vi "UHR-Fleezers Control (host) - 12.2.vi"() -> ()   [LabVIEW 2012] (continued)
            n2466 = VISA Write(VISA resource name=w4106, write buffer=w4105) -> (VISA resource name out=w4102:refnum<visa-resource-name>)  [unwired: 1 in, 2 out]
            n2467 = Concatenate Strings("cvolume" ("string"), "\r") -> (w4103:string)
            n2468 = VISA Write(VISA resource name=w4102, write buffer=w4103) -> (VISA resource name out=w4097:refnum<visa-resource-name>)  [unwired: 1 in, 2 out]
            n2469 = Concatenate Strings("wrun" ("string"), "\r") -> (w4098:string)
            n2470 = VISA Write(VISA resource name=w4097, write buffer=w4098) -> ()  [unwired: 1 in, 3 out]
          }
        }
      }
      event "Flip Green Filter": Value Change {
        n2471 = event-data() -> ()  [unwired: 7 out]
        n2472 = Not(x="Flip Green Filter") -> (.not. x?=w4116:bool)
        n2473 = local write "Flip Green Filter"(w4116) -> ()
        n2474 = flat-sequence {
          tunnel: w4124 -> [w4129]
          tunnel: w4123 -> [w4128]
          tunnel: [w4126] -> w4121
          tunnel: [w4125] -> w4120
          tunnel: [w4131] -> w4119
          tunnel: w4121 -> [w4131]
          tunnel: [w4130] -> w4118
          tunnel: w4120 -> [w4130]
          tunnel: w4119 -> [w4135]
          tunnel: w4118 -> [w4134]
          tunnel: [w4133] -> w4122
          frame #0 {
            n2475 = xnode "Read/Write Control"("FPGA VI Reference In"=w4129, "error in"=w4128, "Green Filter Flipper"=TRUE) -> ("FPGA VI Reference Out"=w4126:T19, "error out"=w4125:errorcluster)
          }
          frame #1 {
            n2476 = Wait (ms)(milliseconds to wait=u32 100) -> ()  [unwired: 1 out]
          }
          frame #2 {
            n2477 = xnode "Read/Write Control"("FPGA VI Reference In"=w4135, "error in"=w4134, "Green Filter Flipper"=FALSE) -> ("error out"=w4133:errorcluster)  [unwired: 1 out]
          }
        }
      }
      event "Pump 1 contents", "Pump 3 contents": Value Change {
        n2478 = event-data() -> ()  [unwired: 7 out]
        n2479 = local read "Pump 1 contents"() -> (→"Pump 1 cont disp":string)
        n2480 = local read "Pump 3 contents"() -> (→"Pump 3 cont disp":string)
      }
      event "Reset Trap Pos. FB": Value Change {
        n2481 = event-data() -> ()  [unwired: 7 out]
        n2482 = xnode "Read/Write Control"("FPGA VI Reference In"=w4141, "error in"=w4140, "Trap Pos. FB Reset"="Reset Trap Pos. FB") -> ()  [unwired: 2 out]
      }
      event "Rem fb disp offset": Value Change {
        n2483 = event-data() -> ()  [unwired: 7 out]
        n2484 = local write "Rem fb disp offset"(FALSE ("Rem fb disp offset")) -> ()
        n2485 = local read "Mean T1 Position (nm)"() -> (w4143:dbl)
        n2486 = local read "FB Trap Pos Offset"() -> (w4144:dbl)
        n2487 = Subtract(x=w4144, y=w4143) -> (x-y=w4142:dbl)
        n2488 = local write "FB Trap Pos Offset"(w4142) -> ()
      }
      event "Threshold (nm)": Value Change {
        n2489 = event-data() -> ()  [unwired: 7 out]
        n2490 = flat-sequence {
          tunnel: w4148 -> [w4156]
          tunnel: w4147 -> [w4155]
          tunnel: [w4149] -> w4146
          tunnel: w4146 -> [w4162]
          frame #0 {
            n2491 = xnode "Read/Write Control"("FPGA VI Reference In"=w4156, "error in"=w4155) -> ("FPGA VI Reference Out"=w4152:T19, "error out"=w4151:errorcluster, "FPGA TTrig Thresh"=w4153:i64)
            n2492 = local read "Threshold stored (nm)"() -> (w4161:dbl)
            n2493 = local read "Threshold (nm)"() -> (w4149:dbl)
            n2494 = local read "AOM X Cal (nm/MHz)"() -> (w4159:dbl)
            n2495 = Subtract(x=w4149, y=w4161) -> (x-y=w4160:dbl)
            n2496 = Divide(x=w4160, y=w4159) -> (x/y=w4157:dbl)
            n2497 = call "IR AOM freq to word.vi"("Frequency In (MHz)"=w4157) -> ("Frequency Word Out (double)"=w4158:dbl)
            n2498 = To Quad Integer(1:w4158) -> (0:w4154:i64)
            n2499 = Add(x=w4153, y=w4154) -> (x+y=w4150:i64)
            n2500 = xnode "Read/Write Control"("FPGA VI Reference In"=w4152, "error in"=w4151, "FPGA TTrig Thresh"=w4150) -> ()  [unwired: 2 out]
          }
          frame #1 {
            "Threshold stored (nm)" <- w4162
          }
        }
      }
      event "FB Trig Integrate": Value Change {
        n2501 = event-data() -> ()  [unwired: 7 out]
        n2502 = local read "FB Trig Integrate"() -> (w4164:u32)
        n2503 = xnode "Read/Write Control"("FPGA VI Reference In"=w4166, "error in"=w4165, "FB Trig Integrate"=w4164) -> ("error out"=w4163:errorcluster)  [unwired: 1 out]
      }
      event "11": Value Change {
        n2504 = event-data() -> ()  [unwired: 7 out]
        n2505 = local read "11"() -> (w4167:bool)
        n2506 = case shown="True" w4167 {
          frame False {
          }
          frame True {
            n2507 = local read "Messages"() -> (w4169:string)
            n2508 = call "Update messages.vi"("Message to add"="You kicked it up to 11!", "Old message string"=w4169) -> ("New message string"=w4170:string)
            n2509 = call <vilib>:"Beep.vi"() -> ()  [unwired: 12 in]
            n2510 = local write "Messages"(w4170) -> ()
          }
        }
      }
      event "Trap Pos. FB ON": Value Change {
        n2511 = event-data() -> ()  [unwired: 7 out]
        n2512 = xnode "Read/Write Control"("FPGA VI Reference In"=w4173, "error in"=w4172, "Force feedback"="Trap Pos. FB ON") -> ()  [unwired: 2 out]
      }
      event "Remove Action Offset": Value Change {
        n2513 = event-data() -> ()  [unwired: 7 out]
        n2514 = local write "Remove Action Offset"(FALSE ("Remove Action Offset")) -> ()
        n2515 = local read "Trap Pos. FB Mult Factor"() -> (w4178:i64)
        n2516 = local read "Trap Pos FB Action"() -> (w4176:i64)
        n2517 = local read "Trap Pos. FB Offset Factor"() -> (w4174:i64)
        n2518 = Multiply(x=w4178, y=w4176) -> (x*y=w4177:i64)
        n2519 = Add(x=w4177, y=w4174) -> (x+y=w4175:i64)
        n2520 = local write "Trap Pos. FB Offset Factor"(w4175) -> ()
        n2521 = xnode "Read/Write Control"("FPGA VI Reference In"=w4181, "error in"=w4180, "Trap Pos. FB Offset Factor"=w4175) -> ()  [unwired: 2 out]
      }
      event "Remove Unwinding Offset": Value Change {
        n2522 = event-data() -> ()  [unwired: 7 out]
        n2523 = local write "Remove Unwinding Offset"(FALSE ("Remove Action Offset")) -> ()
        n2524 = local read "Trap Pos. FB Mult Factor"() -> (w4193:i64)
        n2525 = local read "Trap Pos FB Action"() -> (w4191:i64)
        n2526 = local read "Trap Pos. FB Offset Factor"() -> (w4190:i64)
        n2527 = Multiply(x=w4193, y=w4191) -> (x*y=w4192:i64)
        n2528 = local read "Trap Pos. FB Mult Factor"() -> (w4189:i64)
        n2529 = Add(x=w4192, y=w4190) -> (x+y=w4183:i64)
        n2530 = Multiply(x=32768, y="factor") -> (x*y=w4186:dbl)
        n2531 = Multiply(x=w4186, y=w4189) -> (x*y=w4188:dbl)
        n2532 = Subtract(x=w4183, y=w4188) -> (x-y=w4187:dbl)
        n2533 = To Quad Integer(1:w4187) -> (0:w4182:i64)
        n2534 = xnode "Read/Write Control"("FPGA VI Reference In"=w4196, "error in"=w4195, "Trap Pos. FB Offset Factor"=w4182) -> ()  [unwired: 2 out]
        n2535 = local write "Trap Pos. FB Offset Factor"(w4182) -> ()
      }
      event "Trap Pos. FB Range", "Trap Pos. FB Gains", "Trap Pos. FB Mult Factor", "Trap Pos. FB Offset Factor", "Trap Pos FB Negate Action", "Trap Pos FB Monitor\nT1 or T2", "Differential FB?", "Negate Diff?": Value Change {
        n2536 = event-data() -> ()  [unwired: 7 out]
        n2537 = Unbundle By Name("Trap Pos. FB Gains") -> ("proportional gain (Kc)"=w4199:fxp<+/-,16,8>, "integral gain (Kc*Ts/Ti)"=w4198:fxp<+/-,16,8>, "derivative gain (Kc*Td/Ts)"=w4197:fxp<+/-,16,8>)
        n2538 = local read "Negate Diff?"() -> (w4204:bool)
        n2539 = Unbundle By Name("Trap Pos. FB Range") -> ("output high"=w4202:fxp<+/-,16,1>, "output low"=w4201:fxp<+/-,16,1>)
        n2540 = xnode "Read/Write Control"("FPGA VI Reference In"=w4212, "error in"=w4211, "FB2 output high"=w4202, "FB2 output low"=w4201, "P2"=w4199, "I2"=w4198, "D2"=w4197, "Trap Pos. FB Mult Factor"="Trap Pos. FB Mult Factor", "Trap Pos. FB Offset Factor"="Trap Pos. FB Offset Factor", "Trap Pos FB Negate Action"="Trap Pos FB Negate Action", "Trap Pos FB Monitor T1 or T2"="Trap Pos FB Monitor\nT1 or T2", "AI1 X Scale"="Trap Pos. AI1 X Pre-scale", "Negate Diff?"=w4204, "Diff FB Measurement?"="Differential FB?") -> ()  [unwired: 2 out]
      }
      event "Trap Pos FB SP", "Trap Pos FB SP 2", "Use SP 2": Value Change {
        n2541 = event-data() -> ()  [unwired: 7 out]
        n2542 = Select(t="Trap Pos FB SP 2", s="Use SP 2", f="Trap Pos FB SP") -> (s? t:f=w4213:fxp<+/-,16,1>)
        n2543 = xnode "Read/Write Control"("FPGA VI Reference In"=w4218, "error in"=w4217, "Trap Pos. FB SP"=w4213) -> ()  [unwired: 2 out]
      }
      event "Offset SP2 from SP1": Value Change {
        n2544 = event-data() -> ()  [unwired: 7 out]
        n2545 = local read "Trap Pos FB SP"() -> (w4221:fxp<+/-,16,1>)
        n2546 = Add(x=w4221, y="SP2 Offset") -> (x+y=w4219:fxp<+/-,16,1>)
        n2547 = property on="Trap Pos FB SP 2" class="DigNum (strict)"("Val(Sgnl)"=w4219) -> ()  [unwired: 2 in, 2 out]
        n2548 = local write "Offset SP2 from SP1"(FALSE ("Offset SP2 from SP1")) -> ()
      }
      event "Set Reading to\nSetpoint": Value Change {
        # "This is the actual PID input signal"
        n2549 = event-data() -> ()  [unwired: 7 out]
        n2550 = local write "Set Reading to\nSetpoint"(FALSE ("Set SP to Reading")) -> ()
        n2551 = xnode "Read/Write Control"("FPGA VI Reference In"=w4227, "error in"=w4226) -> ("FPGA VI Reference Out"=w4225:T19, "error out"=w4224:errorcluster, "Trap Pos FB Int-Norm Signal"=w4223:fxp<+/-,16,1>)
        n2552 = local read "Differential FB?"() -> (w4228:bool)
        n2553 = case shown="False" w4228 {
          tunnel: [w4233 w4240] -> w4230
          tunnel: w4223 -> [w4231 w4240]
          frame False {
            n2554 = local read "Trap Pos FB Monitor\nT1 or T2"() -> (w4236:bool)
            n2555 = local read "Trap X AI1 (DMA)"() -> (w4239:T13)
            n2556 = Unbundle By Name(w4239) -> ("Set 1"=w4238:fxp<+/-,16,1>, "Set 2"=w4237:fxp<+/-,16,1>)
            n2557 = Select(t=w4238, s=w4236, f=w4237) -> (s? t:f=w4235:fxp<+/-,16,1>)
            n2558 = Not(x="Set SP Using...") -> (.not. x?=w4232:bool)
            n2559 = Select(t=w4231, s=w4232, f=w4235) -> (s? t:f=w4233:fxp<+/-,16,1>)
          }
          frame True {
          }
        }
        n2560 = xnode "Read/Write Control"("FPGA VI Reference In"=w4225, "error in"=w4224, "Trap Pos. FB SP"=w4230) -> ()  [unwired: 2 out]
        n2561 = local write "Trap Pos FB SP"(w4230) -> ()
      }
      event "Trap Pos. FB Out Scale 2^n": Value Change {
        n2562 = event-data() -> ()  [unwired: 7 out]
        n2563 = Scale By Power Of 2(n="Trap Pos. FB Out Scale 2^n", x=ext 1.0) -> (x*2^n=w4241:ext)
        n2564 = property on="Trap Pos. FB Mult Factor" class="DigNum (strict)"("Val(Sgnl)"=w4241) -> ()  [unwired: 2 in, 2 out]
      }
      event "Trap Pos FB Int Count": Value Change {
        n2565 = event-data() -> ()  [unwired: 7 out]
        n2566 = xnode "Read/Write Control"("FPGA VI Reference In"=w4246, "error in"=w4245, "Trap Pos FB Int Count"="Trap Pos FB Int Count") -> ()  [unwired: 2 out]
      }
      event "Trap pos": Value Change {
        n2567 = event-data() -> ()  [unwired: 7 out]
        n2568 = case shown="True" "Trap pos" {
          frame False {
            n2569 = property on="Trap Delta Graph" class="WFGraph (strict)"("Visible"=TRUE) -> ()  [unwired: 2 in, 2 out]
            n2570 = property on="Saved trap pos" class="WFGraph (strict)"("Visible"=FALSE) -> ()  [unwired: 2 in, 2 out]
          }
          frame True {
            n2571 = property on="Saved trap pos" class="WFGraph (strict)"("Visible"=TRUE) -> ()  [unwired: 2 in, 2 out]
            n2572 = property on="Trap Delta Graph" class="WFGraph (strict)"("Visible"=FALSE) -> ()  [unwired: 2 in, 2 out]
          }
        }
      }
    }
    "error out 2" <- w3101
    n2573 = node-c288() -> ()  [unwired: 2 out]
  }
  n2574 = timed-loop "Rough control of MCL mirror stage (debugging)" {
    tunnel: w52 -> [w4254]
    tunnel: [w4253] -> w268
    timing: w2 -> [_]
    timing-out: [_] -> w1
    stop <- w4253 stop-if-true
    n2575 = node-c288() -> ()  [unwired: 2 out]
    n2576 = case shown="1" "MCL Mode" {
      tunnel: w4254 -> [_ w4257 w4304]
      frame 0, Default {
      }
      frame 1 {
        n2577 = node-c288() -> (w4259:T21)  [unwired: 4 out]
        n2578 = timed-loop "Oscillate MCL mirror" {
          timing: w4259 -> [_]
          timing-out: [_] -> w4258
          tunnel: w4257 -> [w4298]
          i -> [w4297]
          stop <- w4260 stop-if-true
          n2579 = node-c288() -> (w4296:i64)  [unwired: 1 out]
          n2580 = Multiply(x="AO1", y=32767.0) -> (x*y=w4292:dbl)
          n2581 = Multiply(x="AO2", y=32767.0) -> (x*y=w4287:dbl)
          n2582 = Divide(x=w4292, y=10.0) -> (x/y=w4293:dbl)
          n2583 = Divide(x=w4287, y=10.0) -> (x/y=w4288:dbl)
          n2584 = To Word Integer(number=w4293) -> (16bit integer=w4285:i16)
          n2585 = To Word Integer(number=w4288) -> (16bit integer=w4284:i16)
          n2586 = Divide(x=w4296, y=i64 1000) -> (x/y=w4267:dbl)
          n2587 = Multiply(x=w4267, y=w4297) -> (x*y=w4278:dbl)
          n2588 = Multiply(x="Osc. freq. (Hz) 2", y=6.283185307179586) -> (x*y=w4279:dbl)
          n2589 = Multiply(x=w4279, y=w4278) -> (x*y=w4277:dbl)
          n2590 = Sine(x=w4277) -> (sin(x)=w4276:dbl)
          n2591 = Multiply(x=w4276, y="Osc. amp. (V)") -> (x*y=w4274:dbl)
          n2592 = Add(x=w4274, y="Osc. center (V)") -> (x+y=w4272:dbl)
          n2593 = Divide(x=w4272, y=10.0) -> (x/y=w4270:dbl)
          n2594 = Multiply(x=w4270, y=32767.0) -> (x*y=w4265:dbl)
          n2595 = Select(t=w4265, s="Scan axis", f=w4285) -> (s? t:f=w4283:dbl)
          n2596 = Select(t=w4284, s="Scan axis", f=w4265) -> (s? t:f=w4282:dbl)
          n2597 = local read "MCL Mode"() -> (w4264:u16)
          n2598 = Not Equal?(x=w4264, y=u16 1) -> (x != y?=w4261:bool)
          n2599 = local read "Stop All"() -> (w4262:bool)
          n2600 = xnode "Read/Write Control"("FPGA VI Reference In"=w4298, "AO1"=w4283, "AO2"=w4282) -> ()  [unwired: 1 in, 2 out]
          n2601 = Compound Arithmetic op=OR(w4262, w4261) -> (w4260:bool)
          n2602 = node-c288() -> ()  [unwired: 2 out]
        }
        n2603 = node-c288(w4258) -> ()  [unwired: 1 out]
      }
      frame 2 {
        n2604 = case shown="True" "Start Scan" {
          tunnel: w4304 -> [_ w4316]
          frame False {
          }
          frame True {
            n2605 = Subtract(x="End (V)", y="Begin (V)") -> (x-y=w4312:dbl)
            n2606 = Decrement(x="N Points") -> (x-1=w4311:dbl)
            n2607 = Divide(x=w4312, y=w4311) -> (x/y=w4309:dbl)
            n2608 = for {
              N: "N Points" -> [_]
              tunnel: "Begin (V)" -> [w4329]
              tunnel: w4316 -> [w4321]
              tunnel: [w4320] -> w4315 mode=indexing
              tunnel: w4309 -> [w4319]
              tunnel: [w4317] -> w4308 mode=indexing
              i -> [w4328]
              n2609 = Multiply(x=w4319, y=w4328) -> (x*y=w4327:dbl)
              n2610 = Add(x=w4329, y=w4327) -> (x+y=w4324:dbl)
              n2611 = local read "Scan axis"() -> (w4318:bool)
              n2612 = local read "AO1"() -> (w4326:dbl)
              n2613 = local read "AO2"() -> (w4325:dbl)
              n2614 = Select(t=w4324, s=w4318, f=w4326) -> (s? t:f=w4323:dbl)
              n2615 = Select(t=w4325, s=w4318, f=w4324) -> (s? t:f=w4322:dbl)
              n2616 = flat-sequence {
                tunnel: w4323 -> [w4333]
                tunnel: w4322 -> [w4332]
                tunnel: w4321 -> [w4330]
                tunnel: [w4343] -> w4320
                tunnel: [w4342] -> w4317
                frame #0 {
                  w4336 = 10.0 ("y")
                  w4331 = 32767.0 ("y")
                  n2617 = Multiply(x=w4333, y=w4331) -> (x*y=w4339:dbl)
                  n2618 = Multiply(x=w4332, y=w4331) -> (x*y=w4337:dbl)
                  n2619 = Divide(x=w4339, y=w4336) -> (x/y=w4340:dbl)
                  n2620 = Divide(x=w4337, y=w4336) -> (x/y=w4338:dbl)
                  n2621 = To Word Integer(number=w4340) -> (16bit integer=w4334:i16)
                  n2622 = To Word Integer(number=w4338) -> (16bit integer=w4335:i16)
                  n2623 = xnode "Read/Write Control"("FPGA VI Reference In"=w4330, "AO1"=w4334, "AO2"=w4335) -> ()  [unwired: 1 in, 2 out]
                }
                frame #1 {
                  n2624 = Wait (ms)(milliseconds to wait="DAQ Delay (ms)") -> ()  [unwired: 1 out]
                }
                frame #2 {
                  n2625 = local read "Slow mean"() -> (w4343:dbl)
                  n2626 = local read "Sigma"() -> (w4342:dbl)
                }
              }
            }
            n2627 = Bundle("Begin (V)"="Begin (V)", w4309, w4315) -> (→"MCL Scan":cluster{"Begin (V)":dbl, dbl, dbl[]})  [unwired: 1 out]
            n2628 = Bundle("Begin (V)"="Begin (V)", w4309, w4308) -> (→"MCL Scan 2":cluster{"Begin (V)":dbl, dbl, dbl[]})  [unwired: 1 out]
          }
        }
      }
    }
    n2629 = local read "Stop All"() -> (w4253:bool)
    n2630 = node-c288() -> ()  [unwired: 2 out]
  }
  n2631 = timed-loop "Oscillate Trap/AOM (fishing, debugging)" {
    tunnel: w52 -> [w4345]
    tunnel: [w4344] -> w140
    timing: w135 -> [_]
    timing-out: [_] -> w134
    stop <- w4344 stop-if-true
    n2632 = node-c288() -> ()  [unwired: 2 out]
    n2633 = event shown="[0] \"Oscillate Set 1\", \"Fish for Tether\": Value Change" {
      selector: _ -> [_ _ _]
      dyn-events: _ -> [_ _ _]
      timeout: _ -> [_ _ _]
      tunnel: w4345 -> [w4352 _ _]
      tunnel: [FALSE ("Stop All") _ w4941] -> w4344
      event "Oscillate Set 1", "Fish for Tether": Value Change {
        n2634 = event-data() -> ()  [unwired: 6 out]
        n2635 = local read "Oscillate Set 1"() -> (w4351:bool)
        n2636 = Or(x=w4351, y="Fish for Tether") -> (x .or. y?=w4349:bool)
        n2637 = case shown="True" w4349 {
          tunnel: w4352 -> [_ w4355]
          tunnel: "Fish for Tether" -> [_ w4354]
          frame False {
          }
          frame True {
            n2638 = case shown="True" w4354 {
              selector: w4354 -> [w4358 w4364]
              tunnel: [w4358 w4364] -> w4353
              frame False {
              }
              frame True {
                n2639 = local write "Scan axis 2"(TRUE) -> ()
                n2640 = local write "Tether"(FALSE ("Tether")) -> ()
                n2641 = local read "Flow ON during cal?"() -> (w4359:bool)
                n2642 = property on="Trap Delta (MHz)" class="DigNum (strict)"("Val(Sgnl)"="Furthest Delta (MHz)") -> ()  [unwired: 2 in, 2 out]
                n2643 = Or(x="Flow ON during \nfishing?", y=w4359) -> (x .or. y?=w4360:bool)
                n2644 = Wait (ms)(milliseconds to wait=u32 500) -> ()  [unwired: 1 out]
                n2645 = property on="Sample Channel\nFlow" class="Bool (strict)"("Val(Sgnl)"=w4360) -> ()  [unwired: 2 in, 2 out]
              }
            }
            n2646 = node-c288() -> (w4357:T21)  [unwired: 4 out]
            n2647 = timed-loop "Oscillate AOD" {
              timing: w4357 -> [_]
              timing-out: [_] -> w4356
              tunnel: w4355 -> [w4374]
              tunnel: w4353 -> [w4367]
              i -> [w4376]
              stop <- w4373 stop-if-true
              n2648 = node-c288() -> (w4375:i64)  [unwired: 1 out]
              n2649 = flat-sequence {
                tunnel: w4376 -> [w4403]
                tunnel: w4375 -> [w4402]
                tunnel: w4374 -> [w4381]
                tunnel: w4367 -> [w4384]
                tunnel: [w4384] -> w4372
                tunnel: [w4383] -> w4371
                tunnel: [w4380] -> w4370
                tunnel: [w4377] -> w4368
                tunnel: w4372 -> [w4439]
                tunnel: w4371 -> [w4437]
                tunnel: w4370 -> [w4436]
                tunnel: [w4435] -> w4369
                tunnel: w4368 -> [w4434]
                tunnel: [w4511] -> w4373
                tunnel: w4369 -> [w4510]
                frame #0 {
                  n2650 = Divide(x=w4402, y=i64 1000) -> (x/y=w4397:dbl)
                  n2651 = Multiply(x=w4397, y=w4403) -> (x*y=w4399:dbl)
                  n2652 = local read "BD 1 Frequency 2 (MHz)"() -> (w4382:dbl)
                  n2653 = Multiply(x="Osc. freq. (Hz)", y=6.283185307179586) -> (x*y=w4400:dbl)
                  n2654 = Multiply(x=w4400, y=w4399) -> (x*y=w4379:dbl)
                  n2655 = local read "BD 1 Frequency 1 (MHz)"() -> (w4387:dbl)
                  n2656 = local read "BD 2 Frequency 1 (MHz)"() -> (w4386:dbl)
                  n2657 = case shown="True" w4384 {
                    tunnel: w4379 -> [w4409 w4414]
                    tunnel: w4387 -> [_ w4425]
                    tunnel: w4382 -> [_ w4426]
                    tunnel: [w4406 w4420] -> w4385
                    tunnel: [FALSE w4417] -> w4380
                    tunnel: [0.0 w4410] -> w4377
                    frame False {
                      n2658 = Sine(x=w4409) -> (sin(x)=w4407:dbl)
                      n2659 = Multiply(x=w4407, y="Osc. amp. (MHz)") -> (x*y=w4406:dbl)
                    }
                    frame True {
                      n2660 = Cosine(x=w4414) -> (cos(x)=w4429:dbl)
                      n2661 = Subtract(x=w4426, y=w4425) -> (x-y=w4424:dbl)
                      n2662 = Decrement(x=w4429) -> (x-1=w4428:dbl)
                      n2663 = Subtract(x=w4424, y="Closest Delta (MHz)") -> (x-y=w4421:dbl)
                      n2664 = Divide(x=w4428, y=-2.0) -> (x/y=w4422:dbl)
                      n2665 = Multiply(x=w4422, y=w4421) -> (x*y=w4420:dbl)
                      n2666 = local read "Vec Mean of T1 T2"() -> (w4416:dbl[])
                      n2667 = Greater?(x=w4416, y="Stop F (pN)") -> (0:w4418:bool[])
                      n2668 = Or Array Elements(Boolean array=w4418) -> (logical OR=w4417:bool)
                      n2669 = Divide(x=w4414, y=6.283185307179586) -> (x/y=w4413:dbl)
                      n2670 = Round Toward +Infinity(x=w4413) -> (ceil(x): smallest int >= x=w4410:dbl)
                      "Attempts" <- w4410
                      n2671 = Greater?(x=w4410, y="Attempt Limit") -> (0:w4412:bool)
                      n2672 = case shown="True" w4412 {
                        frame False {
                        }
                        frame True {
                          n2673 = local write "Fish for Tether"(FALSE ("Fish for Tether")) -> ()
                          n2674 = call <vilib>:"Beep.vi"() -> ()  [unwired: 3 in, 9 out]
                          n2675 = local read "Messages"() -> (w4431:string)
                          n2676 = call "Update messages.vi"("Message to add"="Tether fishing timeout." ("Messages"), "Old message string"=w4431) -> ("New message string"=→"Messages":string)
                        }
                      }
                    }
                  }
                  n2677 = Select(t=w4387, s="Scan axis 2", f=w4386) -> (s? t:f=w4390:dbl)
                  n2678 = Add(x=w4385, y=w4390) -> (x+y=w4383:dbl)
                  n2679 = Select(t=w4383, s="Scan axis 2", f=w4387) -> (s? t:f=w4393:dbl)
                  n2680 = Select(t=w4386, s="Scan axis 2", f=w4383) -> (s? t:f=w4392:dbl)
                  n2681 = local read "Y RF Frequency Limits (MHz)"() -> (w4388:T16)
                  n2682 = local read "X RF Frequency Limits (MHz)"() -> (w4389:T16)
                  n2683 = local read "BD 1 Frequency 3 (MHz)"() -> (w4396:dbl)
                  n2684 = local read "BD 2 Frequency 2 (MHz)"() -> (w4395:dbl)
                  n2685 = local read "BD 2 Frequency 3 (MHz)"() -> (w4394:dbl)
                  n2686 = call "set RF board frequency - interlace.vi"("Board 2 Frequency Limits"=w4388, "Board 1 Frequency Limits"=w4389, "FPGA VI Reference In"=w4381, "Board 2 Frequency 3 (MHz)"=w4394, "Board 1 Frequency 3 (MHz)"=w4396, "Board 2 Frequency 2 (MHz)"=w4395, "Board 2 Frequency 1 (MHz)"=w4392, "Board 1 Frequency 2 (MHz)"=w4382, "Board 1 Frequency 1  (MHz)"=w4393) -> ()  [unwired: 1 in, 2 out]
                }
                frame #1 {
                  n2687 = And(x=w4439, y=w4436) -> (x .and. y?=w4438:bool)
                  n2688 = case "Only if were fishing and now formed tether" shown="False" w4438 {
                    tunnel: w4437 -> [w4441 w4456]
                    tunnel: [w4440 w4455] -> w4435
                    tunnel: w4434 -> [_ w4451]
                    frame False {
                      n2689 = local read "Fish for Tether"() -> (w4440:bool)
                      n2690 = case shown="False" w4440 {
                        tunnel: w4441 -> [w4442 _]
                        frame False {
                          n2691 = property on="BD 1 Frequency 1 (MHz)" class="DigNum (strict)"("Val(Sgnl)"=w4442) -> ()  [unwired: 2 in, 2 out]
                        }
                        frame True {
                        }
                      }
                    }
                    frame True {
                      w4455 = FALSE ("Fish for Tether")
                      n2692 = call <vilib>:"Beep.vi"() -> ()  [unwired: 3 in, 9 out]
                      n2693 = Number To Decimal String(number=w4451, width (-)=i16 1) -> (decimal integer string=w4449:string)
                      n2694 = Concatenate Strings("Formed tether in ", w4449, " attempt(s)." ("string")) -> (w4446:string)
                      n2695 = local read "Messages"() -> (w4453:string)
                      n2696 = local write "Fish for Tether"(w4455) -> ()
                      n2697 = call "Update messages.vi"("Message to add"=w4446, "Old message string"=w4453) -> ("New message string"=w4452:string)
                      n2698 = local write "Messages"(w4452) -> ()
                      n2699 = Get Date/Time In Seconds() -> (seconds since 1Jan1904=→"Time tether formed":timestamp)
                      n2700 = local read "Flow ON during cal?"() -> (w4443:bool)
                      n2701 = property on="Sample Channel\nFlow" class="Bool (strict)"("Val(Sgnl)"=w4443) -> (error out=w4444:errorcluster)  [unwired: 2 in, 1 out]
                      n2702 = case shown="\"2\", \"3\", \"4\", \"5\", \"6\"" "Then..." {
                        selector: "Then..." -> [_ w4459]
                        tunnel: w4456 -> [w4458 _]
                        tunnel: w4444 -> [_ _]
                        frame "1", Default {
                          n2703 = property on="BD 1 Frequency 1 (MHz)" class="DigNum (strict)"("Val(Sgnl)"=w4458) -> ()  [unwired: 2 in, 2 out]
                        }
                        frame "2", "3", "4", "5", "6" {
                          n2704 = flat-sequence {
                            tunnel: w4459 -> [w4461]
                            frame #0 {
                              n2705 = property on="Trap Delta (MHz)" class="DigNum (strict)"("Val(Sgnl)"="Move to Delta 1 (MHz)") -> ()  [unwired: 2 in, 2 out]
                            }
                            frame #1 {
                              n2706 = case shown="\"5\", \"6\"" w4461 {
                                selector: w4461 -> [w4464 w4474 _]
                                frame "3", "4" {
                                n2707 = flat-sequence {
                                tunnel: w4464 -> [w4465]
                                tunnel: [w4465] -> w4462
                                tunnel: [w4467] -> w4463
                                tunnel: w4462 -> [w4467]
                                tunnel: w4463 -> [w4471]
                                frame #0 {
                                n2708 = property on="Green Laser ON/Interlacing" class="Bool (strict)"("Val(Sgnl)"=TRUE ("Value (Signaling)")) -> ()  [unwired: 2 in, 2 out]
                                }
                                frame #1 {
                                n2709 = Multiply(x="Wait Before Save (s)", y=u32 1000 ("x")) -> (x*y=w4469:u32)
                                n2710 = Wait (ms)(milliseconds to wait=w4469) -> ()  [unwired: 1 out]
                                }
                                frame #2 {
                                n2711 = property on="Start Saving" class="Bool (strict)"("Value"=TRUE ("Start Saving")) -> ()  [unwired: 2 in, 2 out]
                                n2712 = case shown="\"4\"" w4471 {
                                frame Default {
                                }
                                frame "4" {
                                n2713 = property on="Fl. Triggered..." class="Bool (strict)"("Val(Sgnl)"=TRUE ("Value (Signaling)")) -> ()  [unwired: 2 in, 2 out]
                                }
                                }
                                }
                                }
                                }
                                frame "5", "6" {
                                n2714 = stacked-sequence {
                                tunnel: w4474 -> [_ _ _ _ _ _ w4486]
                                frame #0 {
                                n2715 = Replace Array Subset(array=u32[] [0] ("Index Values"), new element="Raster Set Upon Tether", index=0) -> (w4475:u32[])
                                n2716 = property on="Saved AOD Raster Scan Parameter Sets" class="Arr (strict)"("Index Values"=w4475) -> ()  [unwired: 2 in, 2 out]
                                }
                                frame #1 {
                                n2717 = Wait (ms)(milliseconds to wait=u32 500) -> ()  [unwired: 1 out]
                                }
                                frame #2 {
                                n2718 = property on="Load parameters" class="Bool (strict)"("Val(Sgnl)"=TRUE ("Value (Signaling)")) -> ()  [unwired: 2 in, 2 out]
                                n2719 = case shown="True" "Green ON During Raster" {
                                frame False {
                                }
                                frame True {
                                n2720 = property on="Green Laser ON/Interlacing" class="Bool (strict)"("Val(Sgnl)"=TRUE ("Value (Signaling)")) -> ()  [unwired: 2 in, 2 out]
                                }
                                }
                                }
                                frame #3 {
                                n2721 = Wait (ms)(milliseconds to wait=u32 500) -> ()  [unwired: 1 out]
                                }
                                frame #4 {
                                n2722 = property on="Trap Raster Scan" class="Bool (strict)"("Val(Sgnl)"=TRUE ("Value (Signaling)")) -> ()  [unwired: 2 in, 2 out]
                                }
                                frame #5 {
                                n2723 = Wait (ms)(milliseconds to wait=u32 2000) -> ()  [unwired: 1 out]
                                }
                                frame #6 {
                                n2724 = flat-sequence {
                                tunnel: w4486 -> [w4493]
                                frame #0 {
                                n2725 = while {
                                stop <- w4489 stop-if-true
                                n2726 = local read "Raster Scanning..."() -> (w4488:bool)
                                n2727 = local read "Saving..."() -> (w4491:bool)
                                n2728 = Wait (ms)(milliseconds to wait=u32 100) -> ()  [unwired: 1 out]
                                n2729 = Not(x=w4491) -> (.not. x?=w4490:bool)
                                n2730 = Not(x=w4488) -> (.not. x?=w4487:bool)
                                n2731 = And(x=w4490, y=w4487) -> (x .and. y?=w4489:bool)
                                }
                                }
                                frame #1 {
                                n2732 = local read "Tether"() -> (w4494:bool)
                                n2733 = case shown="True" w4494 {
                                tunnel: w4493 -> [_ w4496]
                                frame False {
                                n2734 = property on="Fish for Tether" class="Bool (strict)"("Val(Sgnl)"="Fish again after \nraster break?") -> ()  [unwired: 2 in, 2 out]
                                }
                                frame True {
                                n2735 = stacked-sequence {
                                tunnel: w4496 -> [_ w4500 _ _]
                                frame #0 {
                                n2736 = property on="Trap Delta (MHz)" class="DigNum (strict)"("Val(Sgnl)"="Move to Delta 2 (MHz)") -> ()  [unwired: 2 in, 2 out]
                                n2737 = case shown="True" "Flow ON after\ntether testing?" {
                                frame False {
                                }
                                frame True {
                                n2738 = property on="Sample Channel\nFlow" class="Bool (strict)"("Val(Sgnl)"=TRUE ("Value (Signaling)")) -> ()  [unwired: 2 in, 2 out]
                                }
                                }
                                }
                                frame #1 {
                                n2739 = flat-sequence {
                                tunnel: w4500 -> [w4502]
                                frame #0 {
                                n2740 = Wait (ms)(milliseconds to wait=u32 500) -> ()  [unwired: 1 out]
                                }
                                frame #1 {
                                n2741 = case shown="\"6\"" w4502 {
                                frame Default {
                                }
                                frame "6" {
                                n2742 = property on="Green Laser ON/Interlacing" class="Bool (strict)"("Val(Sgnl)"=TRUE ("Green Laser ON/Interlacing")) -> ()  [unwired: 2 in, 2 out]
                                }
                                }
                                }
                                frame #2 {
                                n2743 = Wait (ms)(milliseconds to wait=u32 500) -> ()  [unwired: 1 out]
                                }
                                frame #3 {
                                n2744 = local write "Start Saving"("Save at end (5, 6)") -> ()
                                }
                                }
                                }
                                frame #2 {
                                n2745 = local read "Bead Sep. Int. Time (s)"() -> (w4508:dbl)
                                n2746 = Multiply(x=w4508, y=1000.0) -> (x*y=w4507:dbl)
                                n2747 = Wait (ms)(milliseconds to wait=w4507) -> ()  [unwired: 1 out]
                                }
                                frame #3 {
                                n2748 = property on="Remove Offset" class="Bool (strict)"("Val(Sgnl)"=TRUE ("Value (Signaling)")) -> ()  [unwired: 2 in, 2 out]
                                }
                                }
                                }
                                }
                                }
                                }
                                }
                                }
                                }
                                frame "2", Default {
                                }
                              }
                            }
                          }
                        }
                      }
                      "Tether" <- "Tether Alarm?"
                    }
                  }
                }
                frame #2 {
                  n2749 = local read "Oscillate Set 1"() -> (w4515:bool)
                  n2750 = local read "Stop All"() -> (w4513:bool)
                  n2751 = Or(x=w4515, y=w4510) -> (x .or. y?=w4512:bool)
                  n2752 = Not(x=w4512) -> (.not. x?=w4514:bool)
                  n2753 = Compound Arithmetic op=OR(w4513, w4514) -> (w4511:bool)
                }
              }
              n2754 = node-c288() -> ()  [unwired: 2 out]
            }
            n2755 = node-c288(w4356) -> ()  [unwired: 1 out]
          }
        }
      }
      event "Fl. Triggered...": Value Change {
        n2756 = event-data() -> ()  [unwired: 7 out]
        n2757 = case shown="True" "Fl. Triggered..." {
          frame False {
          }
          frame True {
            n2758 = node-c288() -> (w4526:T21)  [unwired: 4 out]
            n2759 = timed-loop {
              timing: w4526 -> [_]
              timing-out: [_] -> w4525
              tunnel: "Action" -> [w4534]
              shift-right: [w4531] -> _
              shift-left: u8 255 -> [w4533]
              shift-right: [w4528] -> _
              shift-left: 255 -> [w4530]
              stop <- w4527 stop-if-true
              # "Reset confocal spot"
              n2760 = node-c288() -> ()  [unwired: 2 out]
              n2761 = flat-sequence {
                tunnel: w4534 -> [w4554]
                tunnel: w4533 -> [w4553]
                tunnel: [w4552] -> w4532
                tunnel: w4530 -> [w4539]
                tunnel: [w4538] -> w4529
                tunnel: [w4933] -> w4527
                tunnel: w4532 -> [w4932]
                tunnel: [w4932] -> w4531
                tunnel: [w4931] -> w4528
                tunnel: w4529 -> [w4931]
                frame #0 {
                  n2762 = local read "Delta Fl. 2"() -> (w4551:dbl)
                  n2763 = local read "Delta Fl. 1"() -> (w4546:dbl)
                  n2764 = Multiply(x="Fl. Delta Thresh. (kHz)", y=1000.0) -> (x*y=w4541:dbl)
                  n2765 = Select(t=w4546, s="APD to Watch", f=w4551) -> (s? t:f=w4542:dbl)
                  n2766 = Greater?(x=w4542, y=w4541) -> (0:w4547:bool)
                  n2767 = Or(x="Force Yank", y=w4547) -> (x .or. y?=w4545:bool)
                  n2768 = And(x=w4545, y="Yank when?") -> (x .and. y?=w4543:bool)
                  n2769 = case shown="False" w4543 {
                    tunnel: w4554 -> [w4557 w4758]
                    tunnel: w4553 -> [w4559 w4754]
                    tunnel: [w4559 w4752] -> w4552
                    tunnel: w4542 -> [w4565 _]
                    tunnel: w4541 -> [w4564 _]
                    tunnel: "Force Yank" -> [w4562 _]
                    tunnel: w4539 -> [w4561 w4751]
                    tunnel: [w4560 w4751] -> w4538
                    frame False {
                      n2770 = Negate(x=w4564) -> (-x=w4556:dbl)
                      n2771 = local write "Fl. High"(TRUE ("Fl. High")) -> ()
                      n2772 = Less?(x=w4565, y=w4556) -> (x < y?=w4563:bool)
                      n2773 = Or(x=w4562, y=w4563) -> (x .or. y?=w4558:bool)
                      n2774 = case shown="True" w4558 {
                        tunnel: w4561 -> [w4566 w4576]
                        tunnel: [w4566 w4575] -> w4560
                        tunnel: w4557 -> [_ w4574]
                        frame False {
                        }
                        frame True {
                          n2775 = flat-sequence {
                            tunnel: w4576 -> [w4582]
                            tunnel: w4574 -> [w4579]
                            tunnel: [w4581] -> w4573
                            tunnel: [w4580] -> w4572
                            tunnel: [w4579] -> w4571
                            tunnel: w4570 -> [w4578]
                            tunnel: [w4578] -> w4569
                            tunnel: w4568 -> [w4577]
                            tunnel: [w4577] -> w4567
                            tunnel: [w4653] -> w4575
                            tunnel: w4573 -> [w4653]
                            tunnel: w4572 -> [w4652]
                            tunnel: w4571 -> [w4651]
                            tunnel: w4569 -> [w4650]
                            tunnel: w4567 -> [w4649]
                            frame #0 {
                              n2776 = call <vilib>:"Beep.vi"() -> ()  [unwired: 12 in]
                              n2777 = local write "Waiting"(FALSE ("Waiting")) -> ()
                              n2778 = Increment(x=w4582) -> (x+1=w4581:i32)
                              n2779 = case shown="\"Yank\"" w4579 {
                                tunnel: w4581 -> [_ w4587 _]
                                frame "Alarm", Default {
                                }
                                frame "Yank" {
                                n2780 = flat-sequence {
                                tunnel: w4587 -> [w4590]
                                tunnel: [w4589] -> w4586
                                tunnel: [w4588] -> w4585
                                tunnel: w4586 -> [w4600]
                                tunnel: w4585 -> [w4601]
                                frame #0 {
                                n2781 = local read "Yank Delay (s)"() -> (w4593:dbl)
                                n2782 = local read "N Array El"() -> (w4588:u8)
                                n2783 = Quotient & Remainder(x=w4590, y=w4588) -> (x-y*floor(x/y)=w4589:i32)  [unwired: 1 out]
                                n2784 = Multiply(x=w4593, y=1000.0) -> (x*y=w4591:dbl)
                                n2785 = Wait (ms)(milliseconds to wait=w4591) -> ()  [unwired: 1 out]
                                }
                                frame #1 {
                                n2786 = local read "Yank to which?"() -> (w4595:bool)
                                n2787 = local read "Random Choice"() -> (w4605:bool)
                                n2788 = local read "Yank to Trap Delta (MHz)"() -> (w4598:dbl[])
                                n2789 = local read "Yank to SP"() -> (w4599:dbl[])
                                n2790 = Random Number (0-1)() -> (number: 0 to 1=w4604:dbl)
                                n2791 = Multiply(x=w4601, y=w4604) -> (x*y=w4603:dbl)
                                n2792 = Round Toward -Infinity(1:w4603) -> (0:w4602:dbl)
                                n2793 = Select(t=w4602, s=w4605, f=w4600) -> (s? t:f=w4596:dbl)
                                n2794 = Select(t=w4598, s=w4595, f=w4599) -> (s? t:f=w4597:dbl[])
                                n2795 = Index Array(array=w4597, index=w4596) -> (element=w4594:dbl)
                                n2796 = case shown="True" w4595 {
                                tunnel: w4594 -> [w4606 w4633]
                                frame False {
                                n2797 = flat-sequence {
                                tunnel: w4606 -> [w4607]
                                frame #0 {
                                n2798 = property on="Trap Pos FB SP" class="DigNum (strict)"("Val(Sgnl)"=w4607) -> ()  [unwired: 2 in, 2 out]
                                }
                                frame #1 {
                                n2799 = Wait (ms)(milliseconds to wait=u32 700) -> ()  [unwired: 1 out]
                                }
                                frame #2 {
                                n2800 = local read "Action (%)"() -> (w4612:dbl)
                                n2801 = Absolute Value(x=w4612) -> (abs(x)=w4611:dbl)
                                n2802 = Greater?(x=w4611, y=70.0) -> (0:w4609:bool)
                                n2803 = property on="Remove Action Offset" class="Bool (strict)"("Val(Sgnl)"=w4609) -> ()  [unwired: 2 in, 2 out]
                                }
                                frame #3 {
                                n2804 = for {
                                N: 4 -> [_]
                                n2805 = flat-sequence {
                                frame #0 {
                                n2806 = Wait (ms)(milliseconds to wait=u32 500) -> ()  [unwired: 1 out]
                                }
                                frame #1 {
                                n2807 = local read "Action (%)"() -> (w4618:dbl)
                                n2808 = Absolute Value(x=w4618) -> (abs(x)=w4617:dbl)
                                n2809 = Greater?(x=w4617, y=70.0) -> (0:w4615:bool)
                                n2810 = property on="Remove Action Offset" class="Bool (strict)"("Val(Sgnl)"=w4615) -> ()  [unwired: 2 in, 2 out]
                                }
                                }
                                }
                                }
                                frame #4 {
                                n2811 = Wait (ms)(milliseconds to wait=u32 500) -> ()  [unwired: 1 out]
                                }
                                frame #5 {
                                n2812 = local read "Mean"() -> (w4626:dbl)
                                n2813 = Greater?(x=w4626, y=11.0) -> (0:w4620:bool)
                                n2814 = Not(x=w4620) -> (.not. x?=w4621:bool)
                                n2815 = And(x=w4621, y="Shift confocal") -> (x .and. y?=w4623:bool)
                                n2816 = And(x=w4620, y="Shift confocal") -> (x .and. y?=w4624:bool)
                                n2817 = case shown="True" w4624 {
                                frame False {
                                }
                                frame True {
                                n2818 = local read "Confocal Y 2 (V)"() -> (w4630:dbl)
                                n2819 = local read "Confocal X 2 (V)"() -> (w4629:dbl)
                                n2820 = property on="AO1" class="Slide (strict)"("Val(Sgnl)"=w4630) -> ()  [unwired: 2 in, 2 out]
                                n2821 = property on="AO2" class="Slide (strict)"("Val(Sgnl)"=w4629) -> ()  [unwired: 2 in, 2 out]
                                }
                                }
                                n2822 = case shown="True" w4623 {
                                frame False {
                                }
                                frame True {
                                n2823 = local read "Confocal Y 1 (V)"() -> (w4628:dbl)
                                n2824 = local read "Confocal X 1 (V)"() -> (w4627:dbl)
                                n2825 = property on="AO1" class="Slide (strict)"("Val(Sgnl)"=w4628) -> ()  [unwired: 2 in, 2 out]
                                n2826 = property on="AO2" class="Slide (strict)"("Val(Sgnl)"=w4627) -> ()  [unwired: 2 in, 2 out]
                                }
                                }
                                }
                                frame #6 {
                                n2827 = Wait (ms)(milliseconds to wait=u32 1500) -> ()  [unwired: 1 out]
                                }
                                frame #7 {
                                n2828 = property on="Rem fb disp offset" class="Bool (strict)"("Val(Sgnl)"=TRUE ("Value (Signaling)")) -> ()  [unwired: 2 in, 2 out]
                                }
                                }
                                }
                                frame True {
                                n2829 = flat-sequence {
                                tunnel: w4633 -> [w4634]
                                frame #0 {
                                n2830 = property on="Trap Delta (MHz)" class="DigNum (strict)"("Val(Sgnl)"=w4634) -> ()  [unwired: 2 in, 2 out]
                                }
                                frame #1 {
                                n2831 = Wait (ms)(milliseconds to wait=u32 500) -> ()  [unwired: 1 out]
                                }
                                frame #2 {
                                n2832 = local read "Shift confocal"() -> (w4640:bool)
                                n2833 = local read "Mean"() -> (w4642:dbl)
                                n2834 = Greater?(x=w4642, y=11.0) -> (0:w4639:bool)
                                n2835 = Not(x=w4639) -> (.not. x?=w4638:bool)
                                n2836 = And(x=w4638, y=w4640) -> (x .and. y?=w4636:bool)
                                n2837 = And(x=w4639, y=w4640) -> (x .and. y?=w4637:bool)
                                n2838 = case shown="True" w4637 {
                                frame False {
                                }
                                frame True {
                                n2839 = local read "Confocal Y 2 (V)"() -> (w4646:dbl)
                                n2840 = local read "Confocal X 2 (V)"() -> (w4645:dbl)
                                n2841 = property on="AO2" class="Slide (strict)"("Val(Sgnl)"=w4645) -> ()  [unwired: 2 in, 2 out]
                                n2842 = property on="AO1" class="Slide (strict)"("Val(Sgnl)"=w4646) -> ()  [unwired: 2 in, 2 out]
                                }
                                }
                                n2843 = case shown="True" w4636 {
                                frame False {
                                }
                                frame True {
                                n2844 = local read "Confocal X 1 (V)"() -> (w4643:dbl)
                                n2845 = local read "Confocal Y 1 (V)"() -> (w4644:dbl)
                                n2846 = property on="AO2" class="Slide (strict)"("Val(Sgnl)"=w4643) -> ()  [unwired: 2 in, 2 out]
                                n2847 = property on="AO1" class="Slide (strict)"("Val(Sgnl)"=w4644) -> ()  [unwired: 2 in, 2 out]
                                }
                                }
                                }
                                }
                                }
                                }
                                }
                                }
                                }
                                frame "Image" {
                                n2848 = property on="Confocal Image" class="Bool (strict)"("Val(Sgnl)"=TRUE ("Value (Signaling)")) -> ()  [unwired: 2 in, 2 out]
                                }
                              }
                              n2849 = local write "Fl. High"(FALSE ("Fl. High")) -> ()
                              n2850 = local read "Time (s)"() -> (w4580:dbl)
                            }
                            frame #1 {
                              n2851 = case shown="True" "Auto F Reset" {
                                tunnel: w4652 -> [_ w4657]
                                tunnel: w4651 -> [_ w4656]
                                tunnel: w4650 -> [_ w4655]
                                tunnel: w4649 -> [_ w4654]
                                frame False {
                                }
                                frame True {
                                n2852 = node-c288() -> (w4659:T21)  [unwired: 4 in]
                                n2853 = timed-loop {
                                timing: w4659 -> [_]
                                timing-out: [_] -> w4658
                                tunnel: w4657 -> [w4664]
                                tunnel: w4656 -> [w4663]
                                tunnel: w4655 -> [w4662]
                                tunnel: w4654 -> [w4661]
                                stop <- w4660 stop-if-true
                                n2854 = node-c288() -> ()  [unwired: 1 in, 1 out]
                                n2855 = local read "Fl. Delta Thresh. (kHz)"() -> (w4673:dbl)
                                n2856 = local read "APD to Watch"() -> (w4674:bool)
                                n2857 = local read "Delta Fl. 1"() -> (w4675:dbl)
                                n2858 = local read "Delta Fl. 2"() -> (w4676:dbl)
                                n2859 = local read "Fl. Triggered..."() -> (w4667:bool)
                                n2860 = local read "Stop All"() -> (w4668:bool)
                                n2861 = local read "Reset Force"() -> (w4666:bool)
                                n2862 = Multiply(x=w4673, y=1000.0) -> (x*y=w4671:dbl)
                                n2863 = Not(x=w4667) -> (.not. x?=w4665:bool)
                                n2864 = Select(t=w4675, s=w4674, f=w4676) -> (s? t:f=w4670:dbl)
                                n2865 = Greater?(x=w4670, y=w4671) -> (0:w4669:bool)
                                n2866 = Compound Arithmetic op=OR(w4669, w4668, w4665, w4666) -> (w4660:bool)
                                n2867 = case shown="True" w4660 {
                                tunnel: w4664 -> [_ w4680]
                                tunnel: w4663 -> [_ w4684]
                                tunnel: w4662 -> [_ w4683]
                                tunnel: w4661 -> [_ w4682]
                                frame False {
                                }
                                frame True {
                                n2868 = case shown="\"Yank\"" w4684 {
                                tunnel: w4683 -> [_ w4694]
                                tunnel: w4682 -> [_ w4692]
